vi "Cleaning_Process (SubVI).vi"(10 "Array in":string[](array[string]), 11 "Digital in":refnum<vi>) -> (1 "Array out":string[](array[string]), 2 "Boolean":bool, 3 "empty?":bool)   [LabVIEW 2019]
uses:
  <vilib>/numeric/Random Number (Range) DBL.vi
  d99a476c-56ee-48bc-ad34-ddd67c1d93d9.vi
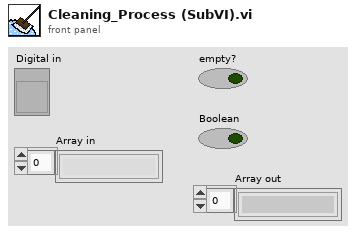
[diagram p1: front panel]
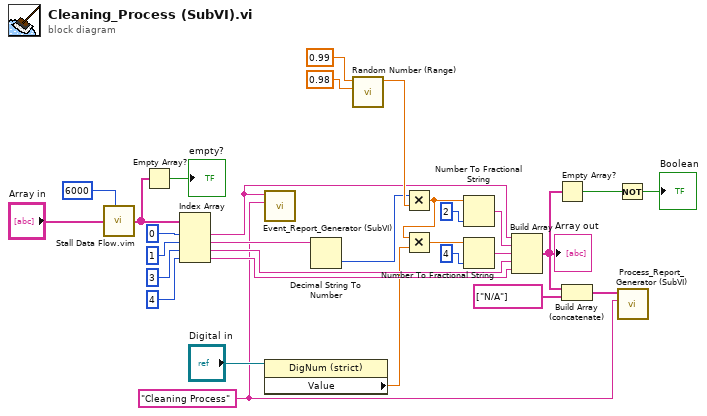
[diagram p0: block diagram]
diagram:
  w6 = "Cleaning Process" ("Process Name")
  n1 = call "Stall Data Flow.vim"("value in"="Array in", "milliseconds to wait"=u32 6000) -> ("value out"=w12:string[])  [unwired: 1 out]
  n2 = Empty Array?(array=w12) -> (empty?=→"empty?":bool)
  n3 = Index Array(array=w12, index #1=0 ("index"), index #2=1 ("index"), index #3=3 ("index"), index #4=4 ("index")) -> (element #1=w7:string, element #2=w15:string, element #3=w27:string, element #4=w28:string)
  n4 = call "Event_Report_Generator (SubVI).vi"("Process Name"=w6, "Booking ID"=w7) -> ()  [unwired: 10 in]
  n5 = property class="DigNum (strict)"(reference="Digital in") -> ("Value"=w21:dbl)  [unwired: 1 in, 2 out]
  n6 = Decimal String To Number(string=w15) -> (number=w2:i32)  [unwired: 2 in, 1 out]
  n7 = call-poly <vilib>:"Random Number (Range).vi"("lower bound (0)"=0.98, "upper bound (100)"=0.99) -> ("number"=w19:dbl)  [unwired: 9 in]
  n8 = Multiply(x=w2, y=w19) -> (x*y=w1:dbl)
  n9 = Multiply(x=w1, y=w21) -> (x*y=w23:dbl)
  n10 = Number To Fractional String(number=w1, precision (6)=i16 2) -> (F-format string=w20:string)  [unwired: 2 in]
  n11 = Number To Fractional String(number=w23, precision (6)=i16 4) -> (F-format string=w24:string)  [unwired: 2 in]
  n12 = Build Array(w7, w20, w24, w27, w28) -> (w4:string[])
  "Array out" <- w4
  n13 = Empty Array?(array=w4) -> (empty?=w29:bool)
  n14 = Build Array (concatenate)(w4, string[] ["N/A"] ("array")) -> (w5:string[])
  n15 = Not(x=w29) -> (.not. x?=→"Boolean":bool)
  n16 = call "Process_Report_Generator (SubVI).vi"("Process Name"=w6, "Process Information"=w5) -> ()  [unwired: 10 in]
